vi "SC_skipstate3_Sub_VI.vi"() -> (2 "Array":dbl[](array[numeric]), 3 "SC States for Weld":dbl[](array[numeric]))   [LabVIEW 2017]
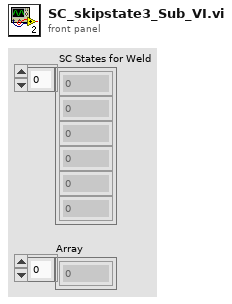
[diagram p1: front panel]
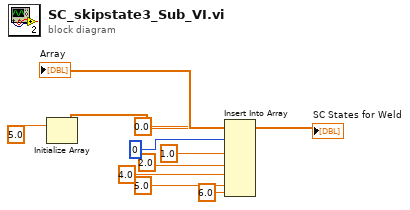
[diagram p0: block diagram]
diagram:
  n1 = Initialize Array(5.0 ("element")) -> (w3:dbl[])  [unwired: 1 in]
  n2 = Insert Into Array(array=w3, index=0, new element #1=0.0 ("new element/subarray"), new element #2=1.0 ("new element/subarray"), new element #3=2.0 ("new element/subarray"), new element #4=4.0 ("new element/subarray"), new element #5=5.0 ("new element/subarray"), new element #6=6.0 ("new element/subarray")) -> (→"SC States for Weld" →"Array":dbl[])
